vi "Write 1.vi"(8 "error in":errorcluster, 10 "1":dbl, 11 "test displayable in":refnum<class "test displayable.lvclass">) -> (0 "error out":errorcluster, 3 "test displayable out":refnum<class "test displayable.lvclass">)   [LabVIEW 2013, in "test displayable.lvclass"]
uses:
  test displayable.lvclass
  test displayable.lvclass/test displayable.ctl
  properties.ctl
  displayable.lvclass
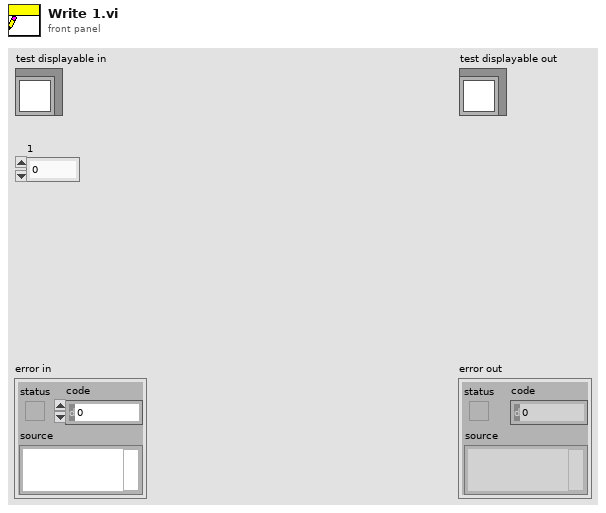
[diagram p1: front panel]
types:
  T1 = typedef "test displayable.lvclass/properties.ctl" = enum16{"1", "2"}
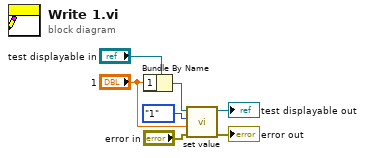
[diagram p0: block diagram]
diagram:
  n1 = Bundle By Name(cluster="test displayable in", "1"="1") -> (w4:refnum<class "test displayable.lvclass">)
  n2 = call "set value.vi"("error in"="error in", "value"="1", "value index"=properties."1" ("props"), "displayable in"=w4) -> ("error out"=→"error out":errorcluster, "displayable out"=→"test displayable out":refnum<class "test displayable.lvclass">)  [unwired: 6 in]
